vi "Cmd.Send.vi"(8 "error in (no error)":errorcluster, 9 "Timeout [ms] (1000)":i32=1000, 10 "Command":string, 11 "connection ID":refnum<k5>) -> (0 "error out":errorcluster, 3 "connection ID out":refnum<k5>)   [LabVIEW 2016]
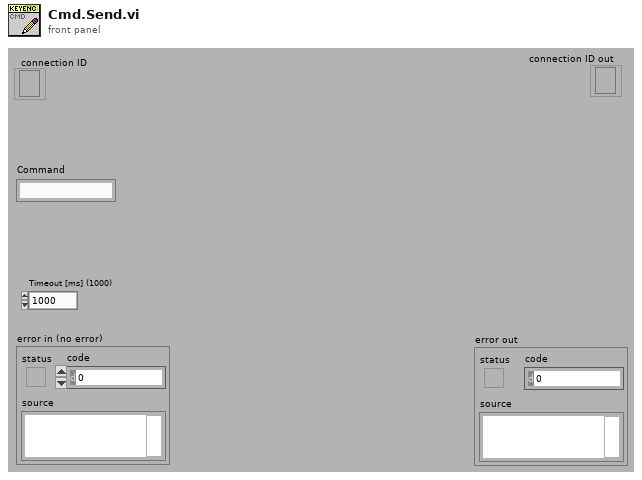
[diagram p1: front panel]
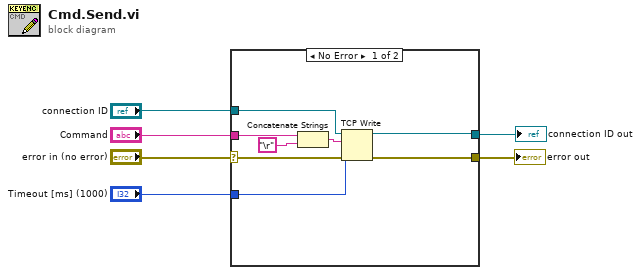
[diagram p0: block diagram]
diagram:
  n1 = case shown="No Error" "error in (no error)" {
    selector: "error in (no error)" -> [w11 w16]
    tunnel: [w7 w16] -> w6
    tunnel: "Timeout [ms] (1000)" -> [w10 _]
    tunnel: "connection ID" -> [w12 w15]
    tunnel: [w9 w15] -> w2
    tunnel: "Command" -> [w14 _]
    frame No Error {
      n2 = Concatenate Strings(w14, "\r") -> (w13:string)
      n3 = TCP Write(connection ID=w12, data in=w13, error in (no error)=w11, 9:w10) -> (connection ID out=w9:refnum<k5>, error out=w7:errorcluster)  [unwired: 1 out]
    }
    frame Error {
    }
  }
  "error out" <- w6
  "connection ID out" <- w2
